vi "CCD LinePatternSetup.vi"(7 "error in":errorcluster, 9 "Shutter Enabled":bool=TRUE, 10 "Exposuretime (s)":dbl=0.5 format="%.2f") -> (0 "error out":errorcluster, 2 "New Image Dimension":i32[](array[numeric]), 3 "Current Setup String":string="ldu,0,256,16;sdu,0,1024,1024;cl0;omrm;sron")   [LabVIEW 2019]
doc: "This VI sets up the CCD camera and assign the setup string to a global variable."
uses:
  Globals and TypeDefs/gDetector.vi
panel:
  in  "Exposuretime(s)":dbl=0.5 format="%.2f"
  in  "Time Delay":u32
  out "Plot Area:Size 2":cluster{"Width":u32, "Height":u32}
  out "Bounds 2":cluster{"Width":u32, "Height":u32}
  out "Position 2":cluster{"Left":i32, "Top":i32}
  out "Plot Area:Size":cluster{"Width":u32, "Height":u32}
  out "Bounds":cluster{"Width":u32, "Height":u32}
  out "Position":cluster{"Left":i32, "Top":i32}
  out "Shot numbers":i32
  in  "stop the continuous shots":bool
  in  "Continuous Shots":bool
  out "1-D Graph":i32[][](graph)
  in  "OK Button":bool
  in  "Tab Control":enum32{"Full Image Shot", "New Image Shot"}(tab)
  out "Proposed Setup String":string="ldu,0,256,16;sdu,0,1024,1024;cl0;omrm;sron"
  in  "Pixels per Block":u16=6 min=1 max=256
  in  "Number of Blocks":u16=25 min=1 max=42
  in  "CCD Lines":cluster{u16, u16}(slide)={1, 1} scale=1.0..256.0
  out "Intensity graph":i32[][](graph)
  out "New Intensity graph":i32[][](graph)
  in  "Initiate CCD":bool
  in  "New Image shot":bool
  out "#PixelOverflow":u32
  out "PixelOverflow":bool
  in  "Full Image Shot":bool
  in  "Set back to array":bool
  in  "Generate color table":bool
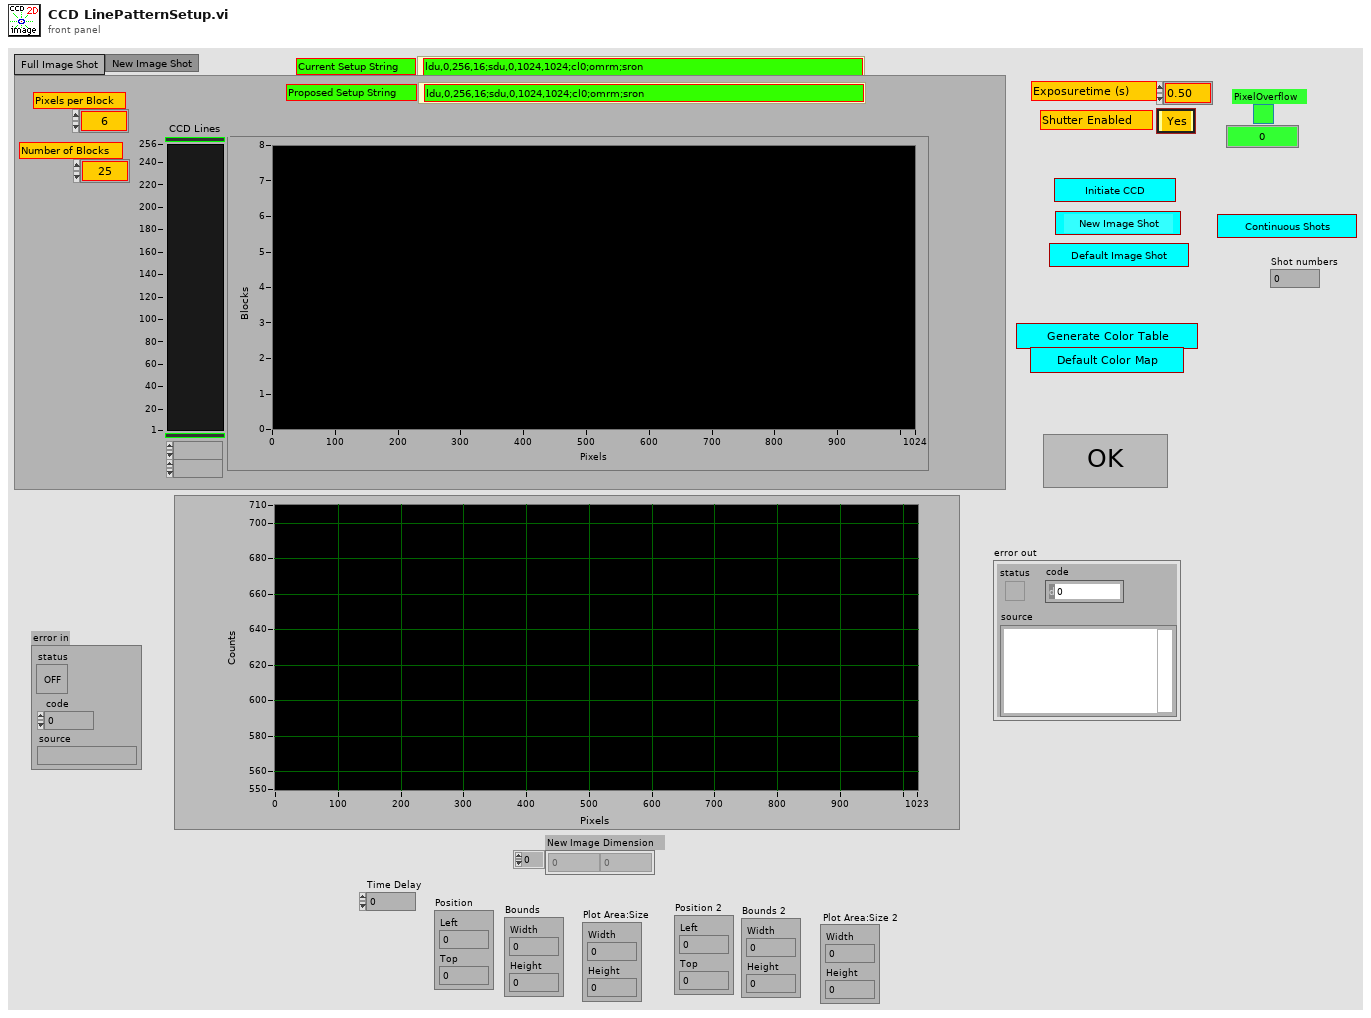
[diagram p1: front panel]
types:
  T1 = typedef "LVPositionTypeDef.ctl" = cluster{"Left":i32, "Top":i32}
  T2 = typedef "LVBoundsTypeDef.ctl" = cluster{"Width":u32, "Height":u32}
  T3 = enum16{"--Quit--", "Init GPIB", "Poll GPIB", "Wait for SRQ", "Clear CCD Parameters", "New CCD Parameters", "Check CCD Command Error"}
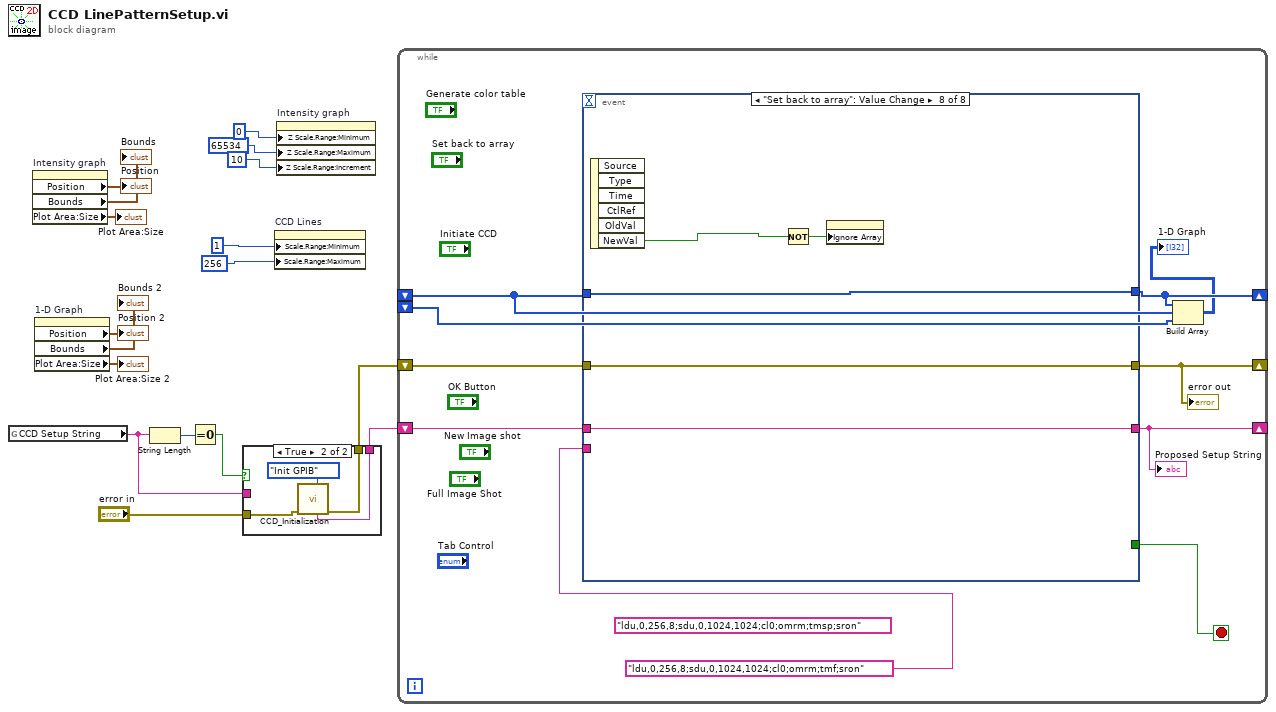
[diagram p0: block diagram]
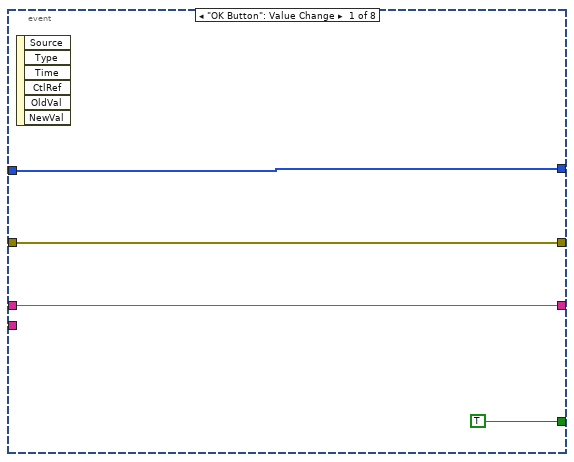
[diagram p3: hidden frame]
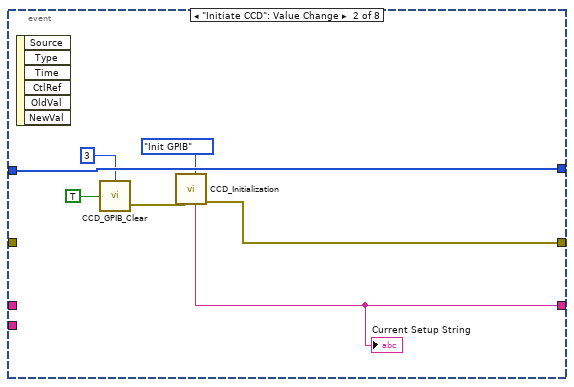
[diagram p4: hidden frame]
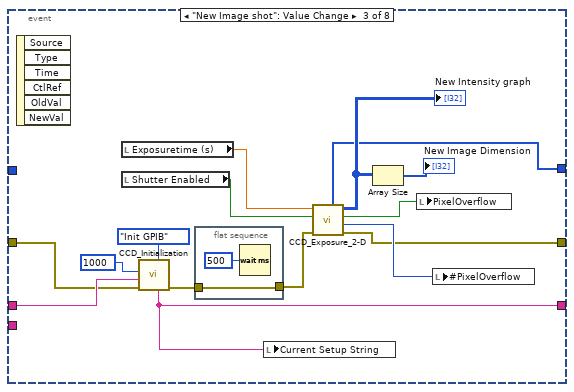
[diagram p5: hidden frame]
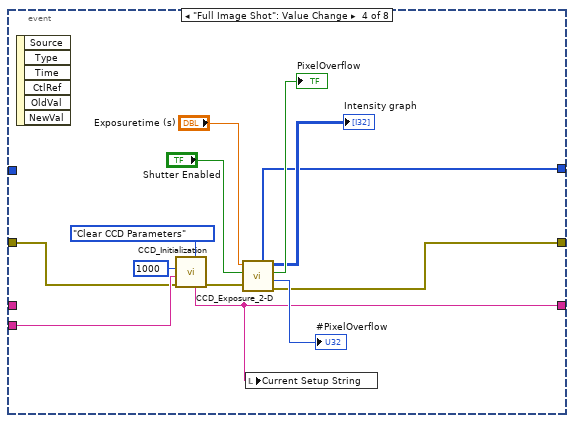
[diagram p6: hidden frame]
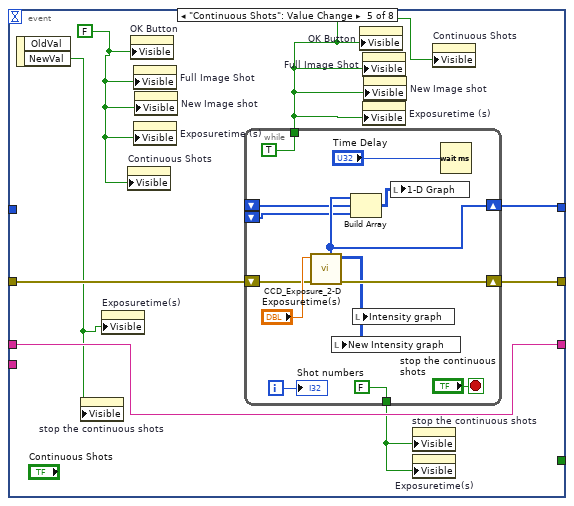
[diagram p7: hidden frame]
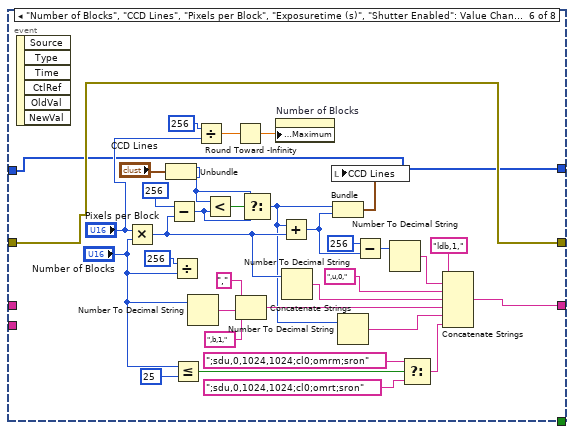
[diagram p8: hidden frame]
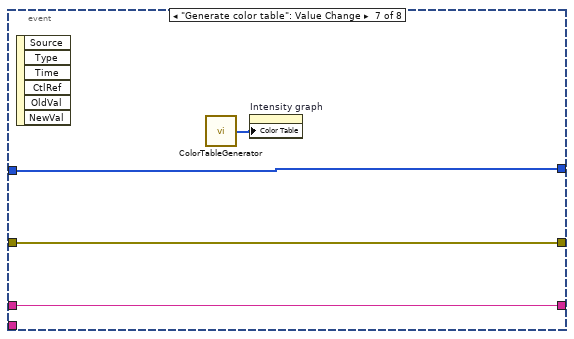
[diagram p9: hidden frame]
diagram:
  n1 = global read "gDetector.vi" "CCD Setup String"() -> (w7:string)
  n2 = property on="Intensity graph" class="IntGraph (strict)"() -> ("Position"=→"Position":T1, "Bounds"=→"Bounds":T2, "Plot Area:Size"=→"Plot Area:Size":T2)  [unwired: 2 in, 2 out]
  n3 = property on="1-D Graph" class="WFGraph (strict)"() -> ("Position"=→"Position 2":T1, "Bounds"=→"Bounds 2":T2, "Plot Area:Size"=→"Plot Area:Size 2":T2)  [unwired: 2 in, 2 out]
  n4 = String Length(string=w7) -> (length=w12:i32)
  n5 = Equal To 0?(x=w12) -> (x = 0?=w11:bool)
  n6 = case shown="True" w11 {
    tunnel: "error in" -> [w19 w23]
    tunnel: [w19 w22] -> w9
    tunnel: [w18 w21] -> w8
    tunnel: w7 -> [w18 _]
    frame False {
    }
    frame True {
      n7 = call "CCD_Initialization.vi"("error in"=w23, "Starting Action"=T3."Init GPIB") -> ("Setup String sent"=w21:string, "error out"=w22:errorcluster)  [unwired: 3 in, 3 out]
    }
  }
  n8 = property on="CCD Lines" class="Slide (strict)"("Scale.Range:Minimum"=u8 1 ("Minimum"), "Scale.Range:Maximum"=u16 256 ("Maximum")) -> ()  [unwired: 2 in, 2 out]
  n9 = property on="Intensity graph" class="IntGraph (strict)"("Z Scale.Range:Minimum"=u32 0 ("Z Minimum"), "Z Scale.Range:Maximum"=u32 65534 ("Z Maximum"), "Z Scale.Range:Increment"=u32 10 ("Z Increment")) -> ()  [unwired: 2 in, 2 out]
  n10 = while {
    shift-right: [w25] -> _
    shift-left: w9 -> [w32]
    shift-right: [w30] -> _
    shift-left: w8 -> [w33]
    shift-right: [w29] -> _
    shift-left: _ -> [w27]
    shift-left: _ -> [w26]
    stop <- w31 stop-if-true
    (unwired) "ldu,0,256,8;sdu,0,1024,1024;cl0;omrm;tmsp;sron"
    n11 = event shown="[7] \"Set back to array\": Value Change" {
      selector: _ -> [_ _ _ _ _ _ _ _]
      dyn-events: _ -> [_ _ _ _ _ _ _ _]
      timeout: _ -> [_ _ _ _ _ _ _ _]
      tunnel: w27 -> [w34 w42 _ _ _ w98 w130 w134]
      tunnel: [w36 w43 w53 w69 w80 w113 w132 w135] -> w30
      tunnel: w33 -> [w36 _ w56 _ w80 _ w132 w135]
      tunnel: "ldu,0,256,8;sdu,0,1024,1024;cl0;omrm;tmf;sron" -> [_ _ _ w71 _ _ _ _]
      tunnel: w32 -> [w37 _ w55 w68 w82 w112 w131 w136]
      tunnel: [w37 w44 w54 w70 w81 w112 w131 w136] -> w25
      tunnel: [TRUE _ _ _ _ _ _ _] -> w31
      tunnel: [w34 w42 w47 w62 w79 w98 w130 w134] -> w29
      event "OK Button": Value Change {
        n12 = event-data() -> ()  [unwired: 1 in, 6 out]
      }
      event "Initiate CCD": Value Change {
        n13 = event-data() -> ()  [unwired: 1 in, 6 out]
        n14 = call "CCD_GPIB_Clear.vi"("#device clearings"=3, "Device Clear?"=TRUE) -> ("error out"=w40:errorcluster)  [unwired: 3 in]
        n15 = call "CCD_Initialization.vi"("error in"=w40, "Starting Action"=T3."Init GPIB") -> ("Setup String sent"=w43:string, "error out"=w44:errorcluster)  [unwired: 3 in, 3 out]
        "Current Setup String" <- w43
      }
      event "New Image shot": Value Change {
        n16 = event-data() -> ()  [unwired: 1 in, 6 out]
        n17 = local read "Exposuretime (s)"() -> (w51:dbl)
        n18 = local read "Shutter Enabled"() -> (w50:bool)
        n19 = call "CCD_Initialization.vi"("milliseconds to wait"=u32 1000, "Setup String"=w56, "error in"=w55, "Starting Action"=T3."Init GPIB") -> ("Setup String sent"=w53:string, "error out"=w46:errorcluster)  [unwired: 1 in, 3 out]
        n20 = flat-sequence {
          tunnel: w46 -> [w61]
          tunnel: [w61] -> w45
          frame #0 {
            n21 = Wait (ms)(milliseconds to wait=u32 500) -> ()  [unwired: 1 out]
          }
        }
        n22 = local write "Current Setup String"(w53) -> ()
        n23 = call "CCD_Exposure_2-D.vi"("error in"=w45, "Shutter Enabled"=w50, "Exposuretime (s)"=w51) -> ("Error Out"=w54:errorcluster, "#PixelOverflow"=w58:u32, "PixelOverflow"=w59:bool, "The Data"=w52:i32[][], "1-D data"=w47:i32[])  [unwired: 2 in, 2 out]
        "New Intensity graph" <- w52
        n24 = Array Size(array=w52) -> (size(s)=→"New Image Dimension":i32[])
        n25 = local write "PixelOverflow"(w59) -> ()
        n26 = local write "#PixelOverflow"(w58) -> ()
      }
      event "Full Image Shot": Value Change {
        n27 = event-data() -> ()  [unwired: 1 in, 6 out]
        n28 = call "CCD_Initialization.vi"("milliseconds to wait"=u32 1000, "Setup String"=w71, "error in"=w68, "Starting Action"=T3."Clear CCD Parameters") -> ("Setup String sent"=w69:string, "error out"=w72:errorcluster)  [unwired: 1 in, 3 out]
        n29 = call "CCD_Exposure_2-D.vi"("error in"=w72, "Shutter Enabled"="Shutter Enabled", "Exposuretime (s)"="Exposuretime (s)") -> ("Error Out"=w70:errorcluster, "#PixelOverflow"=→"#PixelOverflow":u32, "PixelOverflow"=→"PixelOverflow":bool, "The Data"=→"Intensity graph":i32[][], "1-D data"=w62:i32[])  [unwired: 2 in, 2 out]
        n30 = local write "Current Setup String"(w69) -> ()
      }
      event "Continuous Shots": Value Change {
        w76 = FALSE
        n31 = event-data() -> ("NewVal"=w75:bool)  [unwired: 1 in, 1 out]
        n32 = property on="stop the continuous shots" class="Bool"("Visible"=w75) -> ()  [unwired: 2 in, 2 out]
        n33 = property on="Exposuretime(s)" class="DigNum (strict)"("Visible"=w75) -> ()  [unwired: 2 in, 2 out]
        n34 = property on="Continuous Shots" class="Bool"("Visible"=w76) -> ()  [unwired: 2 in, 2 out]
        n35 = property on="OK Button" class="Bool"("Visible"=w76) -> ()  [unwired: 2 in, 2 out]
        n36 = property on="Full Image Shot" class="Bool"("Visible"=w76) -> ()  [unwired: 2 in, 2 out]
        n37 = property on="Exposuretime (s)" class="DigNum (strict)"("Visible"=w76) -> ()  [unwired: 2 in, 2 out]
        n38 = property on="New Image shot" class="Bool"("Visible"=w76) -> ()  [unwired: 2 in, 2 out]
        n39 = while {
          shift-right: [w91] -> w81
          shift-left: w82 -> [w90]
          shift-right: [w88] -> w79
          shift-left: _ -> [w87]
          shift-left: _ -> [w86]
          tunnel: [TRUE] -> w78
          tunnel: [FALSE] -> w77
          i -> [w94]
          stop <- "stop the continuous shots" stop-if-true
          n40 = call "CCD_Exposure_2-D.vi"("error in"=w90, "Exposuretime (s)"="Exposuretime(s)") -> ("Error Out"=w91:errorcluster, "The Data"=w89:i32[][], "1-D data"=w88:i32[])  [unwired: 3 in, 4 out]
          n41 = local write "New Intensity graph"(w89) -> ()
          n42 = Build Array(w88, w87, w86) -> (w85:i32[][])
          n43 = local write "Intensity graph"(w89) -> ()
          n44 = local write "1-D Graph"(w85) -> ()
          n45 = Wait (ms)(milliseconds to wait="Time Delay") -> ()  [unwired: 1 out]
          "Shot numbers" <- w94
        }
        n46 = property on="OK Button" class="Bool"("Visible"=w78) -> ()  [unwired: 2 in, 2 out]
        n47 = property on="Full Image Shot" class="Bool"("Visible"=w78) -> ()  [unwired: 2 in, 2 out]
        n48 = property on="Exposuretime (s)" class="DigNum (strict)"("Visible"=w78) -> ()  [unwired: 2 in, 2 out]
        n49 = property on="New Image shot" class="Bool"("Visible"=w78) -> ()  [unwired: 2 in, 2 out]
        n50 = property on="stop the continuous shots" class="Bool"("Visible"=w77) -> ()  [unwired: 2 in, 2 out]
        n51 = property on="Exposuretime(s)" class="DigNum (strict)"("Visible"=w77) -> ()  [unwired: 2 in, 2 out]
        n52 = property on="Continuous Shots" class="Bool"("Visible"=w78) -> ()  [unwired: 2 in, 2 out]
      }
      event "Number of Blocks", "CCD Lines", "Pixels per Block", "Exposuretime (s)", "Shutter Enabled": Value Change {
        n53 = event-data() -> ()  [unwired: 1 in, 6 out]
        n54 = Multiply(x="Pixels per Block", y="Number of Blocks") -> (x*y=w119:u16)
        n55 = Unbundle("CCD Lines") -> (w105:u16)  [unwired: 1 out]
        n56 = Subtract(x=u16 256 ("Maximum"), y=w119) -> (x-y=w117:u16)
        n57 = Divide(x=u16 256 ("Maximum"), y="Number of Blocks") -> ()  [unwired: 1 out]
        n58 = Less Or Equal?(x="Number of Blocks", y=u8 25) -> (x <= y?=w108:bool)
        n59 = Number To Decimal String(number="Number of Blocks") -> (decimal integer string=w127:string)  [unwired: 1 in]
        n60 = Divide(x=u16 256 ("Maximum"), y="Pixels per Block") -> (x/y=w101:dbl)
        n61 = Less?(x=w105, y=w117) -> (x < y?=w116:bool)
        n62 = Round Toward -Infinity(1:w101) -> (0:w99:dbl)
        n63 = Concatenate Strings(",", w127, ",b,1,") -> (w128:string)
        n64 = Select(t=w105, s=w116, f=w117) -> (s? t:f=w118:u16)
        n65 = property on="Number of Blocks" class="DigNum (strict)"("Data Range:Maximum"=w99) -> ()  [unwired: 2 in, 2 out]
        n66 = Add(x=w118, y=w119) -> (x+y=w120:u16)
        n67 = Number To Decimal String(number=w119) -> (decimal integer string=w125:string)  [unwired: 1 in]
        n68 = Bundle(w118, w120) -> (w114:cluster{u16, u16})  [unwired: 1 in]
        n69 = local write "CCD Lines"(w114) -> ()
        n70 = Number To Decimal String(number=w118) -> (decimal integer string=w96:string)  [unwired: 1 in]
        n71 = Subtract(x=u16 256, y=w120) -> (x-y=w122:u16)
        n72 = Number To Decimal String(number=w122) -> (decimal integer string=w97:string)  [unwired: 1 in]
        n73 = Select(t=";sdu,0,1024,1024;cl0;omrm;sron", s=w108, f=";sdu,0,1024,1024;cl0;omrt;sron") -> (s? t:f=w106:string)
        n74 = Concatenate Strings("ldb,1,", w97, ",u,0,", w125, w128, w96, w106) -> (w113:string)
      }
      event "Generate color table": Value Change {
        n75 = event-data() -> ()  [unwired: 1 in, 6 out]
        n76 = call "ColorTableGenerator.vi"() -> (w133:u32[])
        n77 = property on="Intensity graph" class="IntGraph (strict)"("Color Table"=w133) -> ()  [unwired: 2 in, 2 out]
      }
      event "Set back to array": Value Change {
        n78 = event-data() -> ("NewVal"=w137:bool)  [unwired: 1 in, 5 out]
        n79 = Not(x=w137) -> (.not. x?=w138:bool)
        n80 = property class="IntGraph (strict)"("Ignore Array"=w138) -> ()  [unwired: 2 in, 2 out]
      }
    }
    "Proposed Setup String" <- w30
    "error out" <- w25
    n81 = Build Array(w29, w27, w26) -> (→"1-D Graph":i32[][])
  }
